vi "external cmd - save reply.vi"(0 "Path":path, 7 "reply content":string="reply") -> ()   [LabVIEW 2010]
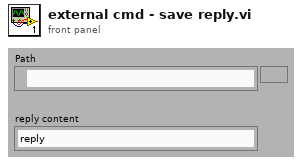
[diagram p1: front panel]
types:
  T1 = enum16{"open", "replace", "create", "open or create", "replace or create", "replace or create with confirmation"}
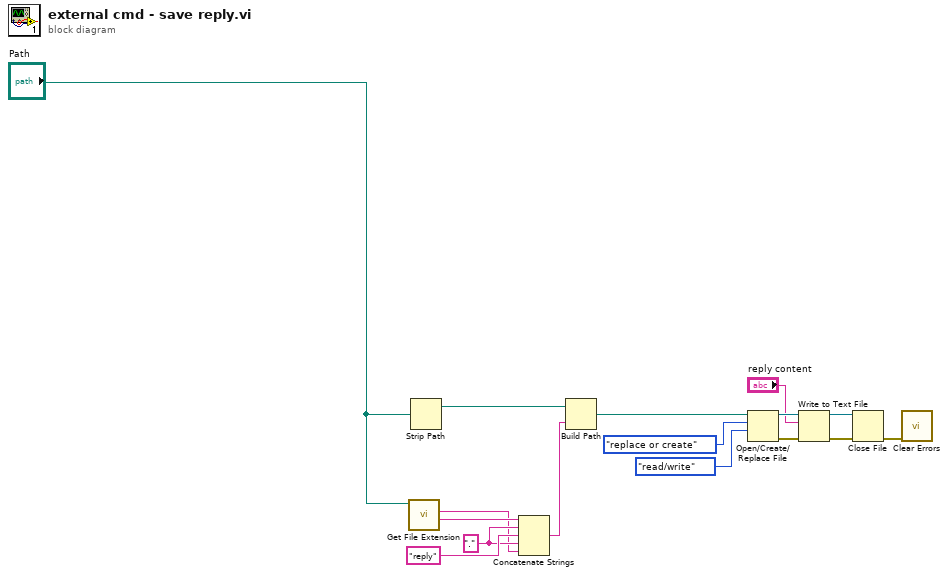
[diagram p0: block diagram]
diagram:
  w2 = "." ("string")
  n1 = call <vilib>:"Get File Extension.vi"("file"="Path") -> ("filename without extension"=w3:string, "lowercase file extension"=w1:string)  [unwired: 7 in, 2 out]
  n2 = Strip Path(path="Path") -> (stripped path=w6:path)  [unwired: 1 out]
  n3 = Concatenate Strings(w3, w2, "reply" ("time format string (%c)"), w2, w1) -> (w7:string)
  n4 = Build Path(base path=w6, name or relative path=w7) -> (appended path=w8:path)
  n5 = Open/Create/Replace File(file path (use dialog)=w8, operation (0:open)=T1."replace or create", access (0:read/write)=enum16{"read/write", "read-only", "write-only"}."read/write") -> (refnum out=w13:refnum<file>, error out=w11:errorcluster)  [unwired: 3 in, 1 out]
  n6 = Write to Text File(file (use dialog)=w13, text="reply content", error in=w11) -> (refnum out=w15:refnum<file>, error out=w14:errorcluster)  [unwired: 1 in, 1 out]
  n7 = Close File(refnum=w15, error in=w14) -> (error out=w16:errorcluster)  [unwired: 1 out]
  n8 = call <vilib>:"Clear Errors.vi"("error in (no error)"=w16) -> ()  [unwired: 6 in, 1 out]
